vi "Read channels.vi"(8 "error in":errorcluster, 11 "CVT configuration in":refnum<class "testmod configuration.lvclass">) -> (0 "error out":errorcluster, 2 "channels":refnum<class "TBM channel.lvclass">[](array[class]), 3 "CVT configuration out":refnum<class "testmod configuration.lvclass">)   [LabVIEW 2013, in "testmod configuration.lvclass"]
uses:
  testmod configuration.lvclass
  <vilib>/NI/Tag Bus Module Framework/channel/TBM channel.lvclass
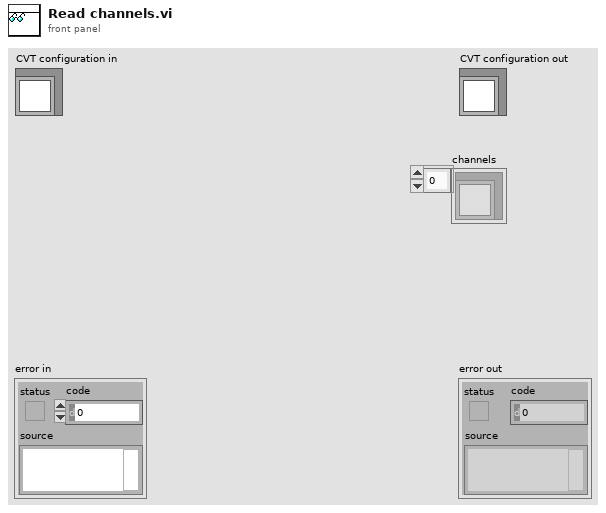
[diagram p1: front panel]
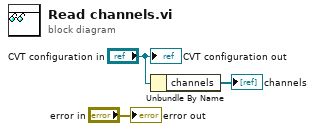
[diagram p0: block diagram]
diagram:
  n1 = Unbundle By Name("CVT configuration in") -> ("channels"=→"channels":refnum<class "TBM channel.lvclass">[])
  "error out" <- "error in"
  "CVT configuration out" <- "CVT configuration in"
